vi "RasPiCompiler.vi"(5 "Compilation Type":T1, 6 "Build Path":path=path "", 7 "Message Box":refnum<vi>, 8 "error in":errorcluster, 11 "VI Path":path) -> (0 "error out":errorcluster, 3 "RasPi Compiler out":refnum<class "RasPi Compiler.lvclass">)   [LabVIEW 2014, in "Raspberry Pi Compatible Compiler for LabVIEW.lvlib" / "RasPi Compiler.lvclass"]
uses:
  RasPi Compiler.lvclass
  Compile and Download App/Custom Controls/CompileType.ctl
  RasPi Compiler.lvclass/RasPi Compiler.ctl
  RasPi_Services/MessageBox/MessageBox.lvclass
  VI Interpreter/Classes/VI Interpreter/VI Interpreter.lvclass
  Raspberry Pi Compatible Compiler for LabVIEW.lvlib
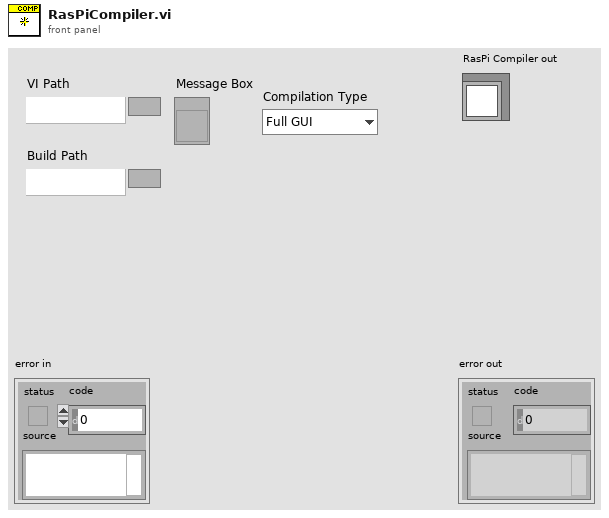
[diagram p1: front panel]
types:
  T1 = typedef "Raspberry Pi Compatible Compiler for LabVIEW.lvlib/CompileType.ctl" = enum16{"Full GUI", "Console App"}
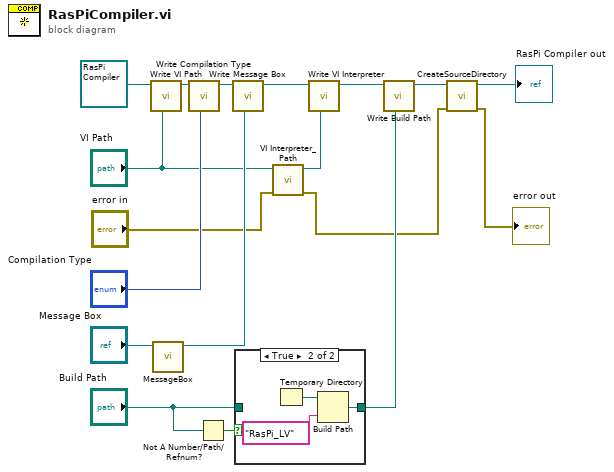
[diagram p0: block diagram]
diagram:
  n1 = call "Write VI Path.vi"("VI Path"="VI Path", "RasPi Compiler in"=refnum<class "RasPi Compiler.lvclass"> refnum) -> ("RasPi Compiler out"=w12:refnum<class "RasPi Compiler.lvclass">)  [unwired: 7 in]
  n2 = call "MessageBox.vi"("Message Box"="Message Box") -> ("MessageBox out"=w10:refnum<class "MessageBox.lvclass">)  [unwired: 9 in, 1 out]
  n3 = call "Write Compilation Type.vi"("Compilation Type"="Compilation Type", "RasPi Compiler in"=w12) -> ("RasPi Compiler out"=w16:refnum<class "RasPi Compiler.lvclass">)  [unwired: 7 in]
  n4 = Not A Number/Path/Refnum?(number/path/refnum="Build Path") -> (NaN/Path/Refnum?=w15:bool)
  n5 = call "Write Message Box.vi"("Message Box"=w10, "RasPi Compiler in"=w16) -> ("RasPi Compiler out"=w8:refnum<class "RasPi Compiler.lvclass">)  [unwired: 7 in]
  n6 = case shown="True" w15 {
    tunnel: "Build Path" -> [w19 _]
    tunnel: [w19 w20] -> w13
    frame False {
    }
    frame True {
      n7 = Temporary Directory() -> (w22:path)
      n8 = Build Path(base path=w22, name or relative path="RasPi_LV") -> (appended path=w20:path)
    }
  }
  n9 = call "VI Interpreter_Path.vi"("error in"="error in", "vi path"="VI Path") -> ("error out"=w1:errorcluster, "VI Interpreter out"=w9:refnum<class "VI Interpreter.lvclass">)  [unwired: 8 in]
  n10 = call "Write VI Interpreter.vi"("VI Interpreter"=w9, "RasPi Compiler in"=w8) -> ("RasPi Compiler out"=w7:refnum<class "RasPi Compiler.lvclass">)  [unwired: 7 in]
  n11 = call "Write Build Path.vi"("Build Path"=w13, "RasPi Compiler in"=w7) -> ("RasPi Compiler out"=w4:refnum<class "RasPi Compiler.lvclass">)  [unwired: 7 in]
  n12 = call "CreateSourceDirectory.vi"("error in"=w1, "RasPi Compiler in"=w4) -> ("error out"=→"error out":errorcluster, "RasPi Compiler out"=→"RasPi Compiler out":refnum<class "RasPi Compiler.lvclass">)  [unwired: 8 in]
